vi "例5.18  DDT数据类型合并信号.vi"() -> ()   [LabVIEW 2017]
panel:
  out "波形图":dynamicdata(graph)
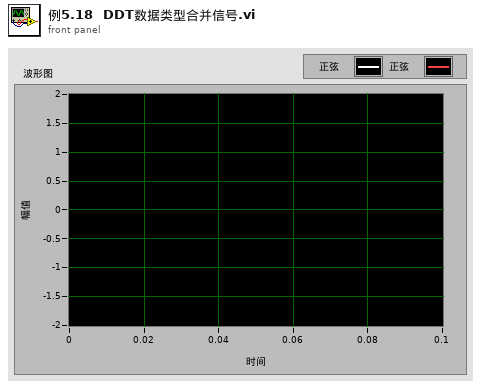
[diagram p1: front panel]
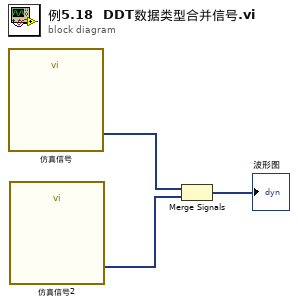
[diagram p0: block diagram]
diagram:
  n1 = call "仿真信号"() -> ("正弦"=w3:dynamicdata)  [unwired: 14 in, 1 out]
  n2 = call "仿真信号2"() -> ("正弦"=w2:dynamicdata)  [unwired: 14 in, 1 out]
  n3 = Merge Signals(w3, w2) -> (→"波形图":dynamicdata)
